vi "Zero IMU.vi"   [LabVIEW 2015]
uses:
  Robot Global Data.vi
  navX-MXP Library/navX-MXP IMU.lvlib
  navX.Library.v2/navX Library v2/navX Library v2.lvlib
types:
  T1 = typedef "navX-MXP IMU.lvlib/navX Device TypeDef.ctl" = cluster{"navX Interface Protocol":T2, "navX Interface Protocol TypeDefs":cluster{"SPIDevRef":T3, "I2CDevRef":T5}, "navX System Information":cluster{"Board Information":T7, "Status":T8, "Offsets":T12}, "navX Common Information":cluster{"Update Rate (4Hz-60Hz)":T13, "refnum name":string, "error":errorcluster}}
  T2 = typedef "navX-MXP IMU.lvlib/navX Interface Protocol.ctl" = enum16{"SPI", "I2C"}
  T3 = typedef "WPI_SPIDevRef.ctl" = cluster{"DevStatus":errorcluster, "Handle":i32, "SPI Bus":T4}
  T4 = typedef "spi_bus.ctl" = enum16{"SPI On-Board, CS0", "SPI On-Board, CS1", "SPI On-Board, CS2", "SPI On-Board, CS3", "SPI MXP", "Invalid"}
  T5 = typedef "WPI_I2CDevRef.ctl" = cluster{"DevStatus":errorcluster, "Device Address":u8, "Handle":i32, "I2C Bus":T6}
  T6 = typedef "i2c_bus.ctl" = enum16{"I2C On-Board", "I2C MXP", "Invalid"}
  T7 = typedef "navX-MXP IMU.lvlib/navX Board Information.ctl" = cluster{"WhoAmI (50 | 0x32)":u8, "Board Revision":u8, "Firmware Major Version":u8, "Firmware Minor Version":u8}
  T8 = typedef "navX-MXP IMU.lvlib/navX Status Data.ctl" = cluster{"Update Rate Hz":u8, "Accelerometer Full-Scale Range":u8, "Gyro Full-Scale Range":u16, "NAVX_OP_STATUS":T9, "NAVX_CAL_STATUS":T10, "NAVX_SELFTEST_STATUS":u8, "NAVX_SENSOR_STATUS":T11}
  T9 = typedef "navX-MXP IMU.lvlib/navX NAVX_OP_STATUS.ctl" = u8
  T10 = typedef "navX-MXP IMU.lvlib/navX NAVX_CAL_STATUS.ctl" = u8
  T11 = typedef "navX-MXP IMU.lvlib/navX NAVX_SENSOR_STATUS.ctl" = cluster{"MOVING":bool, "YAW_STABLE":bool, "MAG_DISTURBANCE":bool, "ALTITUDE_VALID":bool, "SEALEVEL_PRESS_SET":bool, "FUSED_HEADING_VALID":bool}
  T12 = typedef "navX-MXP IMU.lvlib/navX Offsets Data.ctl" = cluster{"Yaw":dbl, "Quat W":dbl, "Quat X":dbl, "Quat Y":dbl, "Quat Z":dbl}
  T13 = typedef "navX-MXP IMU.lvlib/navX Update Rate.ctl" = u8
  T14 = typedef "navX-MXP IMU.lvlib/navX YPRH Data.ctl" = cluster{"Yaw":dbl, "Pitch":dbl, "Roll":dbl, "Heading":dbl}
  T15 = typedef "navX Library v2.lvlib/Z900_navX_DeviceTypeDef.ctl" = cluster{"Interface":cluster{"Protocol":T16, "Update Rate (4Hz-60Hz)":u8, "navX Open TypeDef":variant}, "Notify Packet":refnum<notifier>, "Loop VI Refnum":refnum<vi>, "Ready to Close Occurrence Refnum":refnum<k4>}
  T16 = typedef "navX Library v2.lvlib/Z900_navX_ProtocolTypeDef.ctl" = enum16{"SERIAL", "I2C", "SPI"}
  T17 = cluster{"Yaw":dbl, "Roll":dbl, "Pitch":dbl, "Heading":dbl, "Fused Heading":dbl}
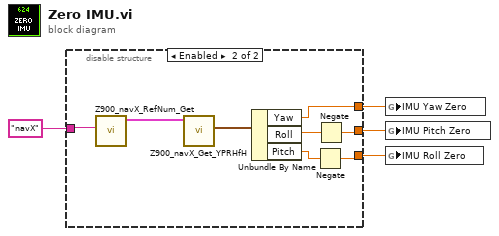
[diagram p0: block diagram]
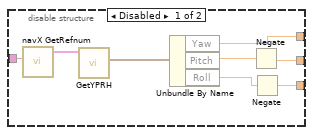
[diagram p2: hidden frame]
diagram:
  n1 = disable-structure shown="Enabled" {
    disable-tunnel: [w10 w13] -> w4
    disable-tunnel: [w9 w14] -> w3
    disable-tunnel: [w8 w17] -> w2
    disable-tunnel: "navX" ("refnum name") -> [w6 w20]
    frame Disabled {
      n2 = call "navX GetRefnum.vi"("refnum name"=w6) -> ("navX Device TypeDef"=w7:T1)  [unwired: 9 in, 1 out]
      n3 = call "GetYPRH.vi"("navX Device TypeDef"=w7) -> ("YPRH"=w5:T14)  [unwired: 8 in, 2 out]
      n4 = Unbundle By Name(w5) -> ("Yaw"=w10:dbl, "Pitch"=w12:dbl, "Roll"=w11:dbl)
      n5 = Negate(x=w12) -> (-x=w8:dbl)
      n6 = Negate(x=w11) -> (-x=w9:dbl)
    }
    frame Enabled {
      n7 = call "Z900_navX_RefNum_Get.vi"("refnum name"=w20) -> ("navX Device"=w19:T15)  [unwired: 9 in, 1 out]
      n8 = call "Z900_navX_Get_YPRHfH.vi"("navX Device"=w19) -> ("YRPHfH"=w18:T17)  [unwired: 7 in, 3 out]
      n9 = Unbundle By Name(w18) -> ("Yaw"=w13:dbl, "Roll"=w16:dbl, "Pitch"=w15:dbl)
      n10 = Negate(x=w15) -> (-x=w14:dbl)
      n11 = Negate(x=w16) -> (-x=w17:dbl)
    }
  }
  n12 = global write "Robot Global Data.vi" "IMU Yaw Zero"(w4) -> ()
  n13 = global write "Robot Global Data.vi" "IMU Pitch Zero"(w2) -> ()
  n14 = global write "Robot Global Data.vi" "IMU Roll Zero"(w3) -> ()
